vi "set_pixel_dwell_time.vi"(8 "error in (no error)":errorcluster, 10 "pixel-dwell time":dbl[unit], 11 "TrajectoryAK101022Resonance in":refnum<class "TrajectoryAK101022Resonance.lvclass">) -> (0 "error out":errorcluster, 3 "TrajectoryAK101022Resonance out":refnum<class "TrajectoryAK101022Resonance.lvclass">)   [LabVIEW 2010, in "TrajectoryAK101022Resonance.lvclass"]
uses:
  TrajectoryAK101022Resonance.lvclass
  FPGAWrapper/GenericFPGAWrapper/GenericFPGAWrapper/GenericFPGAWrapper.lvclass
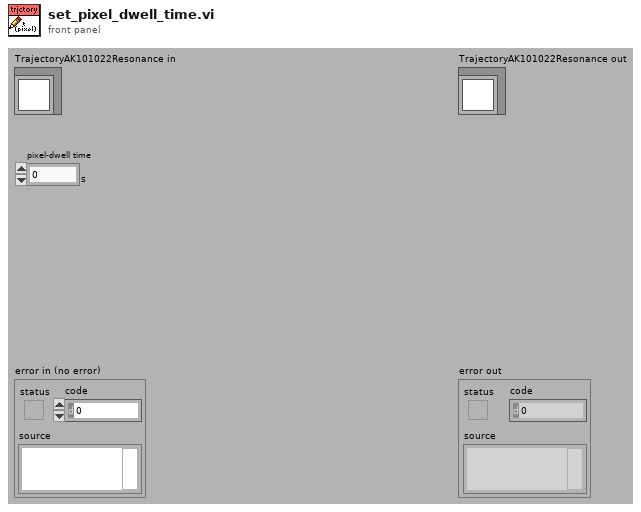
[diagram p1: front panel]
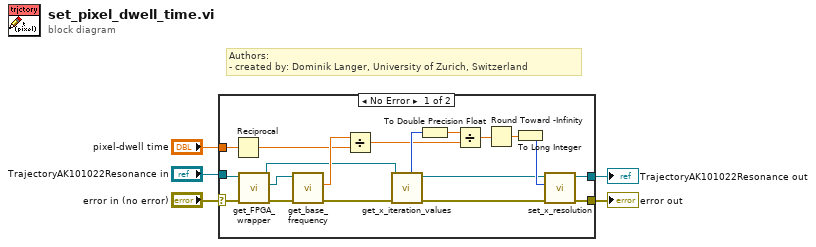
[diagram p0: block diagram]
diagram:
  # "Authors: \n- created by: Dominik Langer, University of Zurich, Switzerland"
  n1 = case shown="No Error" "error in (no error)" {
    selector: "error in (no error)" -> [w19 w26]
    tunnel: [w11 w26] -> w4
    tunnel: [w10 w25] -> w2
    tunnel: "TrajectoryAK101022Resonance in" -> [w9 w25]
    tunnel: "pixel-dwell time" -> [w22 _]
    frame No Error {
      n2 = Reciprocal(x=w22) -> (1/x=w20:dbl[unit])
      n3 = call-dynamic "get_FPGA_wrapper.vi"("error in (no error)"=w19, "TrajectoryMG100122GenericFPGA in"=w9) -> ("error out"=w24:errorcluster, "GenericFPGAWrapper.lvclass"=w23:refnum<class "GenericFPGAWrapper.lvclass">, "TrajectoryMG100122GenericFPGA out"=w8:refnum<class "TrajectoryAK101022Resonance.lvclass">)  [unwired: 7 in]
      n4 = call-dynamic "get_base_frequency.vi"("error in (no error)"=w24, "GenericFPGAWrapper in"=w23) -> ("error out"=w18:errorcluster, "base frequency"=w21:dbl[unit])  [unwired: 7 in, 1 out]
      n5 = Divide(x=w21, y=w20) -> (x/y=w15:dbl)
      n6 = call-dynamic "get_x_iteration_values.vi"("error in (no error)"=w18, "TrajectoryAK101022Resonance in"=w8) -> ("error out"=w7:errorcluster, "TrajectoryAK101022Resonance out"=w6:refnum<class "TrajectoryAK101022Resonance.lvclass">, "scan segment [iterations]"=w17:u16)  [unwired: 4 in, 3 out]
      n7 = To Double Precision Float(number=w17) -> (double precision float=w16:dbl)
      n8 = Divide(x=w16, y=w15) -> (x/y=w14:dbl)
      n9 = Round Toward -Infinity(1:w14) -> (0:w13:dbl)
      n10 = To Long Integer(number=w13) -> (32bit integer=w12:i32)
      n11 = call-dynamic "set_x_resolution.vi"("error in (no error)"=w7, "x resolution"=w12, "TrajectoryAK101022Resonance in"=w6) -> ("error out"=w11:errorcluster, "TrajectoryAK101022Resonance out"=w10:refnum<class "TrajectoryAK101022Resonance.lvclass">)  [unwired: 7 in]
    }
    frame Error {
    }
  }
  "error out" <- w4
  "TrajectoryAK101022Resonance out" <- w2
